vi "Elevator In Range.vi"(9 "Height Tolerance":dbl, 10 "Target Height":dbl, 11 "Actual Height":dbl) -> (3 "In Range":bool)   [LabVIEW 2017]
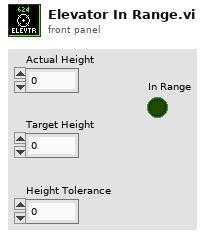
[diagram p1: front panel]
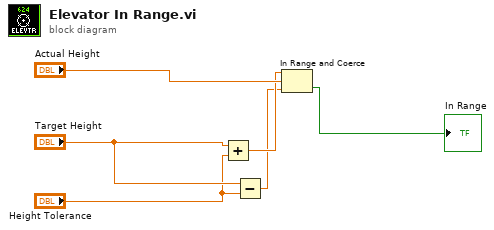
[diagram p0: block diagram]
diagram:
  n1 = Add(x="Target Height", y="Height Tolerance") -> (x+y=w5:dbl)
  n2 = Subtract(x="Target Height", y="Height Tolerance") -> (x-y=w2:dbl)
  n3 = In Range and Coerce(upper limit=w5, x="Actual Height", lower limit=w2) -> (In Range?=→"In Range":bool)  [unwired: 1 out]
